vi "CompilerProcessPulses.vi"(0 "Pulse Seq In":T1[](array[typedef])=[{"enabled"=FALSE, "string"="", "time"=0.0, "step"=0.0, "dio"=0.0, "count"=0.0, "trigger"=0.0, "AO"=0.0}]) -> (1 "Counts used":u8, 2 "# VFG pulses":i32, 3 "Pulse Seq Out":T1[](array[typedef]))   [LabVIEW 2019]
uses:
  SinglePulse.ctl
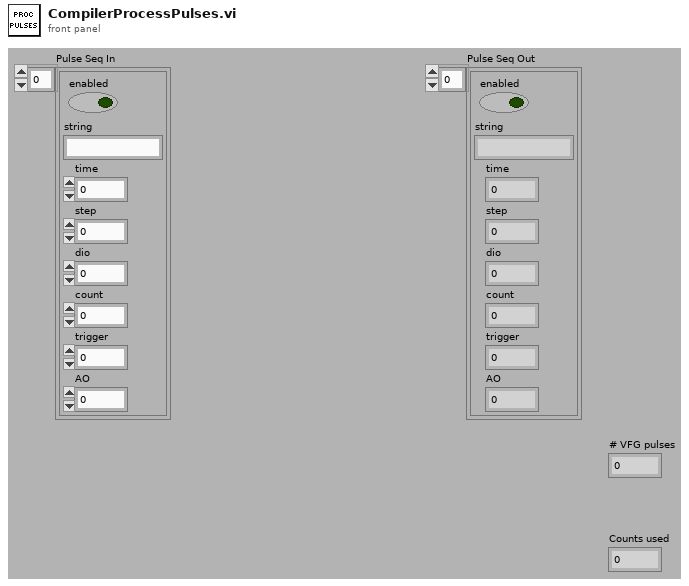
[diagram p1: front panel]
types:
  T1 = typedef "SinglePulse.ctl" = cluster{"enabled":bool, "string":string, "time":dbl, "step":dbl, "dio":dbl, "count":dbl, "trigger":dbl, "AO":dbl}
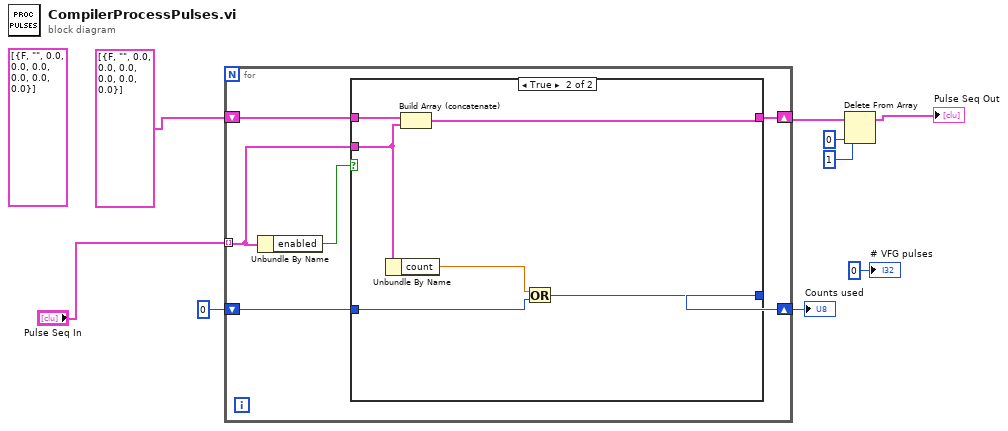
[diagram p0: block diagram]
diagram:
  (unwired) T1[] [{"enabled"=FALSE, "string"="", "time"=0.0, "step"=0.0, "dio"=0.0, "count"=0.0, "trigger"=0.0, "AO"=0.0}] ("Pulse Seq In 2")
  n1 = for {
    tunnel: "Pulse Seq In" -> [w12] mode=indexing
    shift-right: [w13] -> w4
    shift-left: T1[] [{"enabled"=FALSE, "string"="", "time"=0.0, "step"=0.0, "dio"=0.0, "count"=0.0, "trigger"=0.0, "AO"=0.0}] ("Pulse Seq In 2") -> [w14]
    shift-right: [w10] -> w8
    shift-left: u8 0 -> [w11]
    n2 = Unbundle By Name(w12) -> ("enabled"=w15:bool)
    n3 = case shown="True" w15 {
      tunnel: w14 -> [w17 w23]
      tunnel: [w17 w22] -> w13
      tunnel: w12 -> [_ w19]
      tunnel: w11 -> [w16 w21]
      tunnel: [w16 w20] -> w10
      frame False {
      }
      frame True {
        n4 = Unbundle By Name(w19) -> ("count"=w18:dbl)
        n5 = Build Array (concatenate)(w23, w19) -> (w22:T1[])
        n6 = Or(x=w18, y=w21) -> (x .or. y?=w20:i32)
      }
    }
  }
  "Counts used" <- w8
  n7 = Delete From Array(array=w4, length=1, index=0) -> (array with subset deleted=→"Pulse Seq Out":T1[])  [unwired: 1 out]
  "# VFG pulses" <- 0 ("# VFG pulses")
